vi "uintLCM.vi"(8 "Error in (no error)":errorcluster, 10 "Int2 in":refnum<class "UintClass.lvclass">, 11 "Int1 in":refnum<class "UintClass.lvclass">) -> (0 "Error out":errorcluster, 1 "Timing":u32, 3 "LCM(Int1,Int2)":refnum<class "UintClass.lvclass">)   [LabVIEW 2011, in "UintClass.lvclass"]
uses:
  UintClass.lvclass
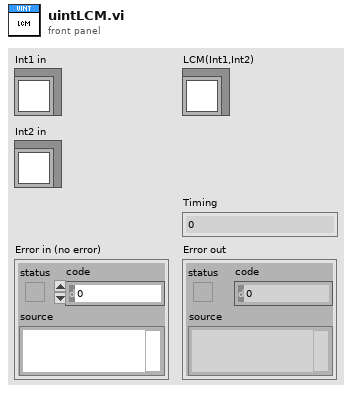
[diagram p1: front panel]
types:
  T1 = typedef "UintClass.lvclass/enumBase.ctl" = u16
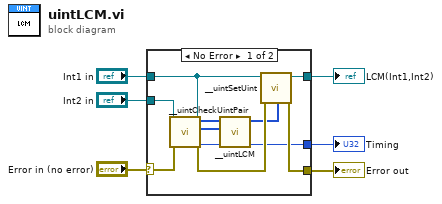
[diagram p0: block diagram]
diagram:
  n1 = case shown="No Error" "Error in (no error)" {
    selector: "Error in (no error)" -> [w16 w18]
    tunnel: "Int1 in" -> [w15 _]
    tunnel: "Int2 in" -> [w17 _]
    tunnel: [w12 _] -> w3
    tunnel: [w13 w18] -> w1
    tunnel: [w7 _] -> w2
    frame No Error {
      n2 = call "__uintCheckUintPair.vi"("Error in (no error)"=w16, "Uint2 in"=w17, "Uint1 in"=w15) -> ("Error out"=w14:errorcluster, "Uint2 out"=w9:u8[], "Uint1 out"=w10:u8[], "Base out"=w11:T1)  [unwired: 5 in]
      n3 = call "__uintLCM.vi"("Base (decimal)"=w11, "Uint2 in"=w9, "Uint1 in"=w10) -> ("Timing"=w7:u32, "LCM(Int1,Int2)"=w8:u8[])  [unwired: 7 in]
      n4 = call "__uintSetUint.vi"("Error in (no error)"=w14, 10:"Uint in"=w8, 11:"Uint in"=w15) -> ("Error out"=w13:errorcluster, "Uint out"=w12:refnum<class "UintClass.lvclass">)  [unwired: 7 in]
    }
    frame Error {
    }
  }
  "Error out" <- w1
  "Timing" <- w2
  "LCM(Int1,Int2)" <- w3
